vi "Start Module.vi"(8 "error in (no error)":errorcluster, 11 "Run as Singleton? (F)":bool) -> (0 "error out":errorcluster, 1 "Wait for Event Sync?":bool, 2 "Device Under Test_Cloneable_DQMH Broadcast Events":T1, 3 "Module ID":i32)   [LabVIEW 2015, in "Device Under Test_Cloneable_DQMH.lvlib"]
doc: "Launches the Module Main.vi.\n_____\nBased on Delacor QMH Project Template 2.0.0.62.\n____\nDelacor QMH Thermal Chamber Examples 4.0.0.21\nCopyright (c) 2018, Delacor"
uses:
  Device Under Test_Cloneable_DQMH.lvlib
  Broadcast Events--cluster.ctl
  Did Init Argument--cluster.ctl
  Status Updated Argument--cluster.ctl
  Error Reported Argument--cluster.ctl
  Stop Argument--cluster.ctl
  Update DUT Status Argument--cluster.ctl
  Get Module Execution Status Argument--cluster.ctl
  Module Running State--enum.ctl
  <vilib>/Delacor/Delacor QMH/Libraries/Cloneable Module Admin_class/Delacor_lib_QMH_Cloneable Module Admin.lvclass
  <vilib>/Delacor/Delacor QMH/Libraries/Cloneable Module Admin_class/Delacor_lib_QMH_Cloneable Module Admin.lvclass/Delacor_lib_QMH_Cloneable Module Admin.ctl
  <vilib>/Delacor/Delacor QMH/Libraries/Module Admin_class/Delacor_lib_QMH_Module Admin.lvclass/Delacor_lib_QMH_Module Admin.ctl
  <vilib>/Delacor/Delacor QMH/Libraries/Cloneable Module Admin_class/Delacor_lib_QMH_Set Module ID.vi
  <vilib>/Delacor/Delacor QMH/Libraries/Module Admin_class/Delacor_lib_QMH_Set External Launch.vi
  <vilib>/Utility/error.llb/Error Cluster From Error Code.vi
  <vilib>/ErrorRing/Error Ring.xnode
  Clone Registration/Clone Registration.lvlib
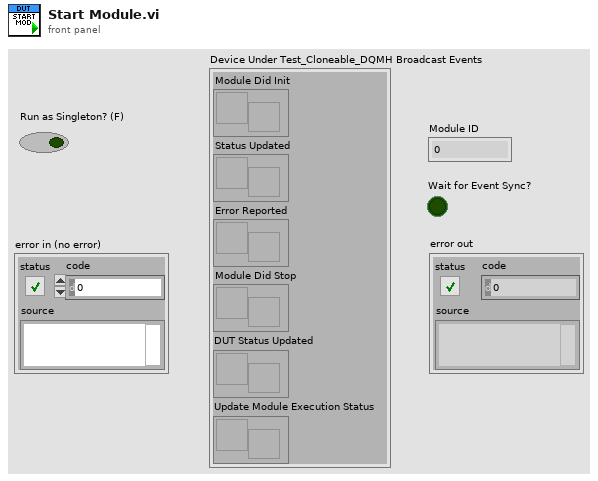
[diagram p1: front panel]
types:
  T1 = typedef "Device Under Test_Cloneable_DQMH.lvlib/Broadcast Events--cluster.ctl" = cluster{"Module Did Init":refnum<user-event>, "Status Updated":refnum<user-event>, "Error Reported":refnum<user-event>, "Module Did Stop":refnum<user-event>, "DUT Status Updated":refnum<user-event>, "Update Module Execution Status":refnum<user-event>}
  T2 = typedef "Device Under Test_Cloneable_DQMH.lvlib/Module Running State--enum.ctl" = enum16{"Not Running", "Running as Cloneable", "Running as Singleton"}
  T3 = enum32{"Bad", "Idle", "Run top level", "Running"}
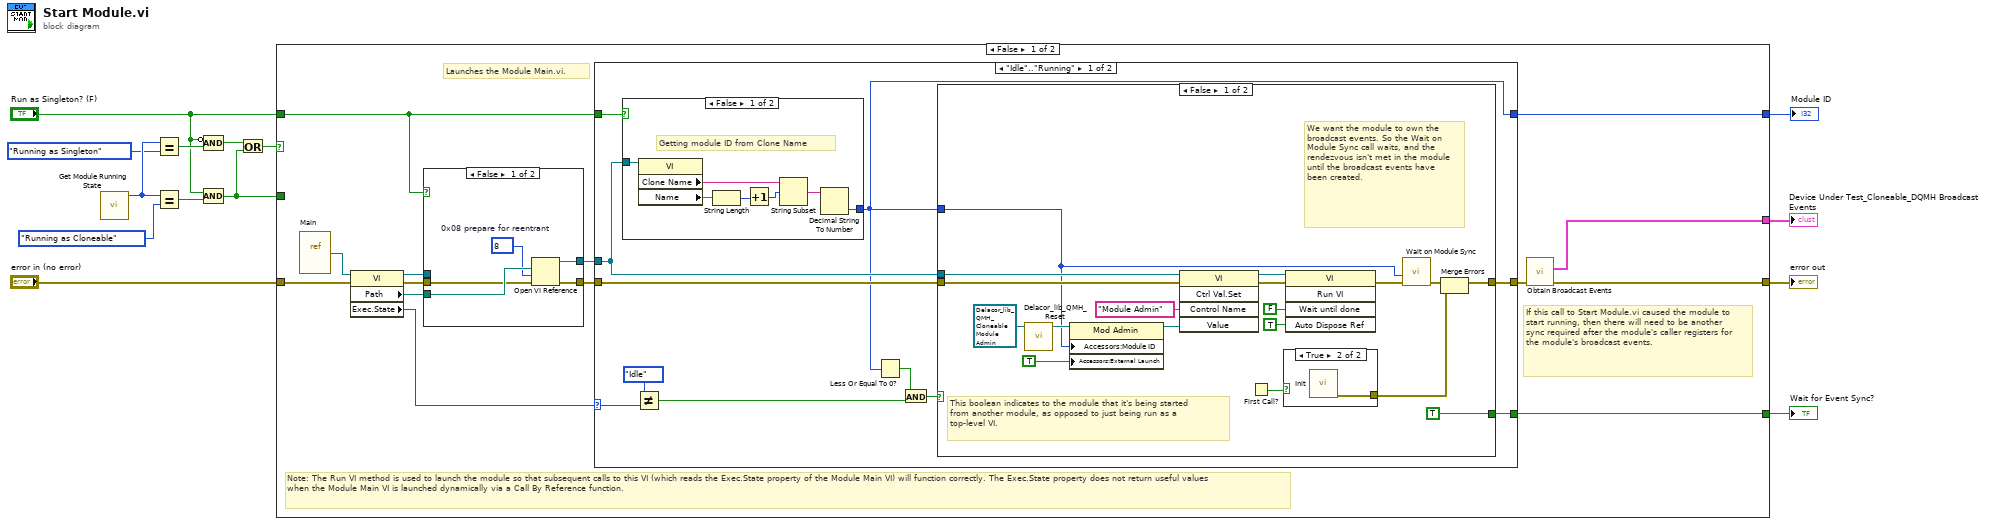
[diagram p0: block diagram]
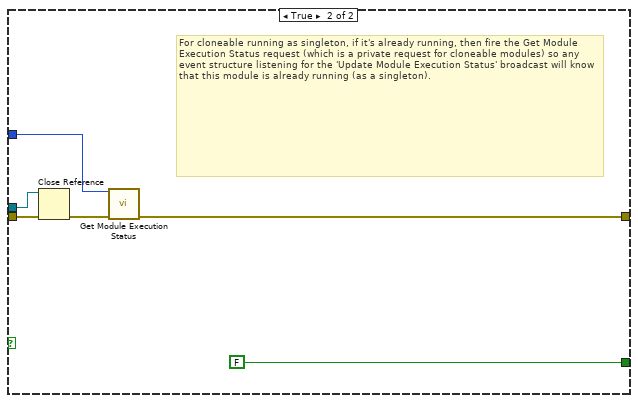
[diagram p4: hidden frame]
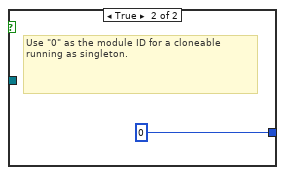
[diagram p5: hidden frame]
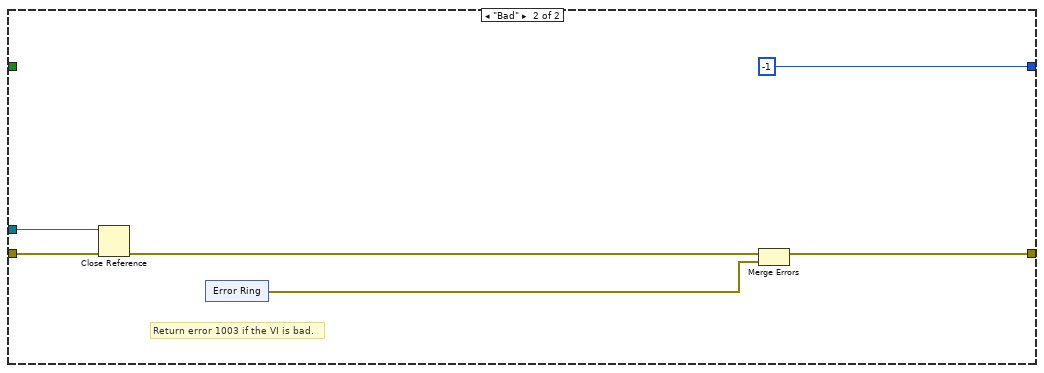
[diagram p6: hidden frame]
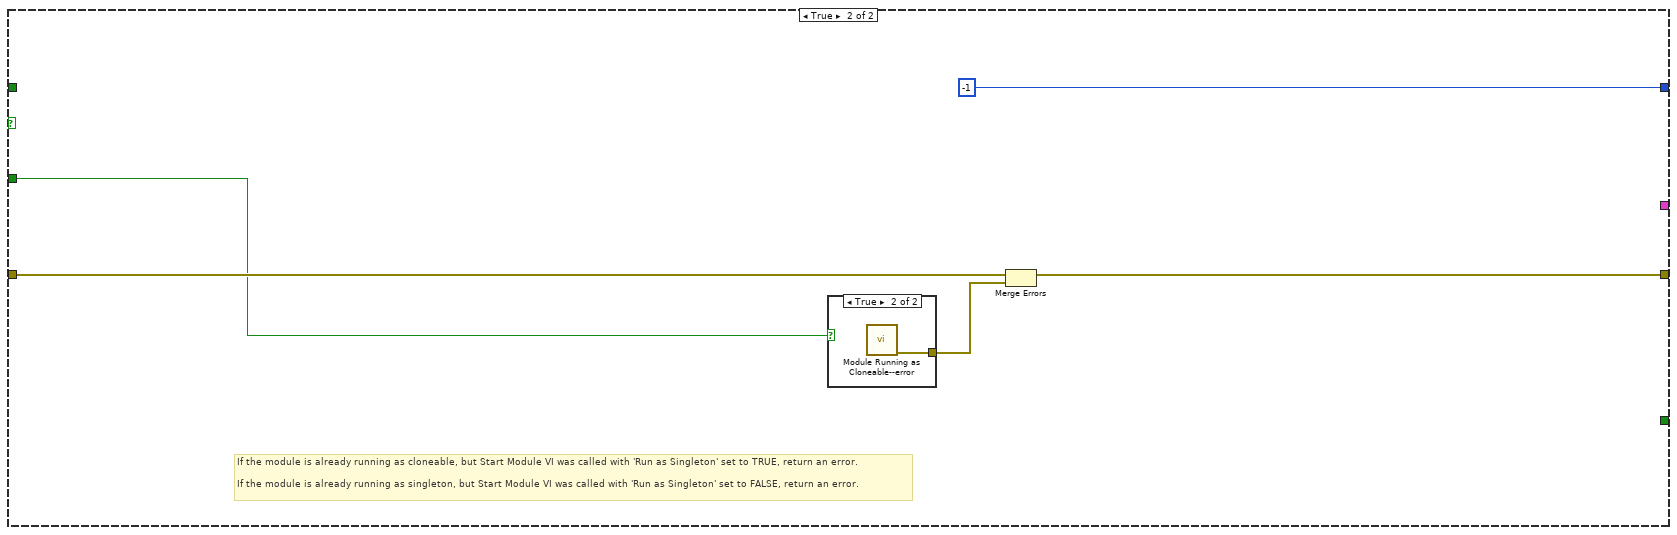
[diagram p7: hidden frame]
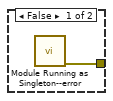
[diagram p8: hidden frame]
diagram:
  n1 = call "Get Module Running State.vi"() -> ("Module Running State"=w9:T2)  [unwired: 11 in]
  n2 = Equal?(x=w9, y=Module_Running_State--enum."Running as Singleton") -> (x = y?=w6:bool)
  n3 = Equal?(x=w9, y=Module_Running_State--enum."Running as Cloneable") -> (x = y?=w5:bool)
  n4 = Compound Arithmetic op=AND(invert "Run as Singleton? (F)", w6) -> (w4:bool)
  n5 = Compound Arithmetic op=AND("Run as Singleton? (F)", w5) -> (w2:bool)
  n6 = Or(x=w4, y=w2) -> (x .or. y?=w3:bool)
  n7 = case shown="False" w3 {
    tunnel: "error in (no error)" -> [w28 w93]
    tunnel: [w26 w92] -> w13
    tunnel: [w25 _] -> w12
    tunnel: [w24 _] -> w11
    tunnel: [w20 -1] -> w10
    tunnel: w2 -> [_ w91]
    tunnel: "Run as Singleton? (F)" -> [w16 _]
    frame False {
      # "Note: The Run VI method is used to launch the module so that subsequent calls to this VI (which reads the Exec.State property of the Module Main VI) will function correctly. The Exec.State property does not return useful values when the Module Main VI is launched dynamically via a Call By Reference function."
      # "If this call to Start Module.vi caused the module to start running, then there will need to be another sync required after the module's caller registers for the module's broadcast events."
      # "Launches the Module Main.vi."
      n8 = vi-ref "Main.vi"() -> (w19:refnum<vi>)
      n9 = property class="VI"(reference=w19, error in=w28) -> (reference out=w15:refnum<vi>, error out=w22:errorcluster, "Path"=w23:path, "Exec.State"=w17:T3)
      n10 = case shown="False" w16 {
        tunnel: w23 -> [w33 _]
        tunnel: w22 -> [w32 w35]
        tunnel: [w31 w35] -> w21
        tunnel: [w29 w34] -> w18
        tunnel: w15 -> [_ w34]
        frame False {
          w30 = 8  # 0x08 prepare for reentrant
          n11 = Open VI Reference(vi path=w33, options=w30, error in (no error)=w32) -> (vi reference=w29:refnum<vi>, error out=w31:errorcluster)  [unwired: 3 in]
        }
        frame True {
        }
      }
      n12 = case shown="\"Idle\"..\"Running\"" w17 {
        selector: w17 -> [w41 _]
        tunnel: w21 -> [w46 w85]
        tunnel: w18 -> [w44 w84]
        tunnel: [w43 w82] -> w27
        tunnel: [w45 _] -> w24
        tunnel: [w36 -1] -> w20
        tunnel: w16 -> [w42 _]
        frame "Idle".."Running" {
          n13 = case shown="False" w42 {
            tunnel: w44 -> [w78 _]
            tunnel: [w72 0] -> w36
            frame False {
              # "Getting module ID from Clone Name"
              n14 = property class="VI"(reference=w78) -> ("Clone Name"=w75:string, "Name"=w74:string)  [unwired: 1 in, 2 out]
              n15 = String Length(string=w74) -> (length=w76:i32)
              n16 = Increment(x=w76) -> (x+1=w77:i32)
              n17 = String Subset ("Getting module ID from Clone Name")(string=w75, offset (0)=w77) -> (substring=w73:string)  [unwired: 1 in]
              n18 = Decimal String To Number(string=w73) -> (number=w72:i32)  [unwired: 2 in, 1 out]
            }
            frame True {
              # "Use \"0\" as the module ID for a cloneable running as singleton."
            }
          }
          n19 = Not Equal?(x=T3."Idle", y=w41) -> (x != y?=w39:bool)
          n20 = Less Or Equal To 0?(x=w36) -> (x <= 0?=w38:bool)
          n21 = And(x=w38, y=w39) -> (x .and. y?=w37:bool)
          n22 = case shown="False" w37 {
            tunnel: w46 -> [w64 w71]
            tunnel: [TRUE FALSE] -> w45
            tunnel: w44 -> [w57 w70]
            tunnel: [w53 w67] -> w43
            tunnel: w36 -> [w47 w68]
            frame False {
              # "We want the module to own the broadcast events. So the Wait on Module Sync call waits, and the rendezvous isn't met in the module until the broadcast events have been created."
              # "This boolean indicates to the module that it's being started from another module, as opposed to just being run as a top-level VI."
              n23 = call-dynamic "Delacor_lib_QMH_Reset.vi"("Mod Admin in"=refnum<class "Delacor_lib_QMH_Cloneable Module Admin.lvclass"> refnum) -> ("Mod Admin out"=w51:refnum<class "Delacor_lib_QMH_Cloneable Module Admin.lvclass">)  [unwired: 9 in, 1 out]
              n24 = property class="Mod Admin"(reference=w51, "Accessors:Module ID"=w47, "Accessors:External Launch"=TRUE) -> (reference out=w50:refnum<class "Delacor_lib_QMH_Cloneable Module Admin.lvclass">)  [unwired: 1 in, 1 out]
              n25 = invoke class="VI" method="Ctrl Val.Set"(reference=w57, error in=w64, "Control Name"="Module Admin", "Value"=w50) -> (reference out=w55:refnum<vi>, error out=w54:errorcluster)  [unwired: 1 in, 3 out]
              n26 = First Call?() -> (First Call?: T/F=w56:bool)
              n27 = case shown="True" w56 {
                tunnel: [_ w65] -> w52
                frame False {
                }
                frame True {
                  n28 = call "Init.vi"() -> ("error out"=w65:errorcluster)  [unwired: 8 in, 3 out]
                }
              }
              n29 = invoke class="VI" method="Run VI"(reference=w55, error in=w54, "Wait until done"=FALSE ("Wait Until Done"), "Auto Dispose Ref"=TRUE ("Auto Dispose Reference")) -> (error out=w61:errorcluster)  [unwired: 1 in, 4 out]
              n30 = call "Wait on Module Sync.vi"("error in (no error)"=w61, "Module ID"=w47) -> ("error out"=w60:errorcluster)  [unwired: 9 in]
              n31 = Merge Errors(w60, w52) -> (w53:errorcluster)
            }
            frame True {
              # "For cloneable running as singleton, if it's already running, then fire the Get Module Execution Status request (which is a private request for cloneable modules) so any event structure listening for the 'Update Module Execution Status' broadcast will know that this module is already running (as a singleton)."
              n32 = Close Reference(reference=w70, error in (no error)=w71) -> (error out=w69:errorcluster)
              n33 = call "Get Module Execution Status.vi"("error in (no error)"=w69, "Module ID"=w68) -> ("error out"=w67:errorcluster)  [unwired: 9 in]
            }
          }
        }
        frame "Bad" {
          # "Return error 1003 if the VI is bad."
          n34 = Close Reference(reference=w84, error in (no error)=w85) -> (error out=w83:errorcluster)
          n35 = xnode "Error Ring"() -> ("error out"=w81:errorcluster)
          n36 = Merge Errors(w83, w81) -> (w82:errorcluster)
        }
      }
      n37 = call "Obtain Broadcast Events.vi"("error in (no error)"=w27) -> ("error out"=w26:errorcluster, "Device Under Test_Cloneable_DQMH Broadcast Events"=w25:T1)  [unwired: 9 in]
    }
    frame True {
      # "If the module is already running as cloneable, but Start Module VI was called with 'Run as Singleton' set to TRUE, return an error.\n\nIf the module is already running as singleton, but Start Module VI was called with 'Run as Singleton' set to FALSE, return an error."
      n38 = case shown="True" w91 {
        tunnel: [w95 w96] -> w90
        frame False {
          n39 = call "Module Running as Singleton--error.vi"() -> ("error out"=w95:errorcluster)  [unwired: 11 in]
        }
        frame True {
          n40 = call "Module Running as Cloneable--error.vi"() -> ("error out"=w96:errorcluster)  [unwired: 11 in]
        }
      }
      n41 = Merge Errors(w93, w90) -> (w92:errorcluster)
    }
  }
  "error out" <- w13
  "Device Under Test_Cloneable_DQMH Broadcast Events" <- w12
  "Wait for Event Sync?" <- w11
  "Module ID" <- w10
